vi "initindexstime.vi"(0 "object in":refnum<class "interface.lvclass">, 5 "error in (no error)":errorcluster) -> (14 "object out":refnum<class "interface.lvclass">, 19 "error out":errorcluster)   [LabVIEW 2016, in "interface.lvclass"]
uses:
  interface.lvclass
  <vilib>/Utility/config.llb/NI_LVConfig.lvlib
  <vilib>/Utility/config.llb/Read Key (String).vi
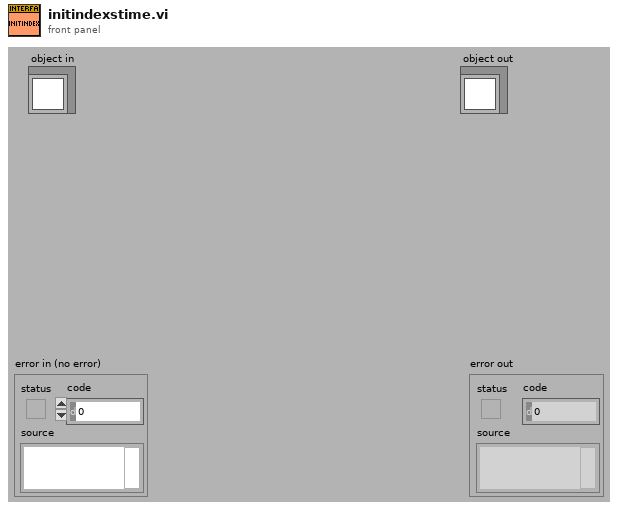
[diagram p1: front panel]
types:
  T1 = cluster{"CODMn":string, "CODCr":string, "DO":string, "铜":string, "PH":string, "氨氮":string, "比电导率":string, "水温":string, "COD":string, "浊度":string, "总氮":string, "总磷":string, "叶绿素a":string, "藻密度":string, "水位":string, "流速":string, "瞬时流量":string, "累积流量":string, "亚硝酸盐":string, "硫化物":string, "ORP":string, "铅":string, "镉":string, "锌":string, "镍":string, "锰":string, "汞":string, "气温":string, "气压":string, "风速":string, "风向":string, "盐度":string, "磷酸盐":string, "硝氮":string, "氟化物":string, "挥发酚":string, "氯化物":string}
  T2 = cluster{"氨氮仪器参数索引起始时间":string, "总磷仪器参数索引起始时间":string, "总氮仪器参数索引起始时间":string, "CODMn仪器参数索引起始时间":string, "CODCr仪器参数索引起始时间":string, "DO仪器参数索引起始时间":string, "PH仪器参数索引起始时间":string, "比电导率仪器参数索引起始时间":string, "水温仪器参数索引起始时间":string, "浊度仪器参数索引起始时间":string, "叶绿素a仪器参数索引起始时间":string, "藻密度仪器参数索引起始时间":string, "ORP仪器参数索引起始时间":string, "氟化物仪器参数索引起始时间":string, "挥发酚仪器参数索引起始时间":string}
  T3 = typedef "LVDateTimeRec.ctl" = cluster{"秒数的小数部分":dbl, "秒":i32, "分":i32, "时":i32, "日":i32, "月":i32, "年":i32, "天数（周）":i32, "天数（年）":i32, "DST":i32}
  T4 = cluster{"氨氮报警信息索引起始时间":string, "总磷报警信息索引起始时间":string, "总氮报警信息索引起始时间":string, "CODMn报警信息索引起始时间":string, "CODCr报警信息索引起始时间":string, "DO报警信息索引起始时间":string, "PH报警信息索引起始时间":string, "比电导率报警信息索引起始时间":string, "水温报警信息索引起始时间":string, "浊度报警信息索引起始时间":string, "叶绿素报警信息索引起始时间":string, "系统报警信息索引起始时间":string, "氟化物报警信息索引起始时间":string, "挥发酚报警信息索引起始时间":string}
  T5 = cluster{"氨氮零点核查索引起始时间":string, "总磷零点核查索引起始时间":string, "总氮零点核查索引起始时间":string, "CODMn零点核查索引起始时间":string, "CODCr零点核查索引起始时间":string, "亚硝酸盐零点核查索引起始时间":string, "硫化物零点核查索引起始时间":string, "ORP零点核查索引起始时间":string, "氟化物零点核查索引起始时间":string, "挥发酚零点核查索引起始时间":string}
  T6 = cluster{"氨氮加标回收索引起始时间":string, "总磷加标回收索引起始时间":string, "总氮加标回收索引起始时间":string, "CODMn加标回收索引起始时间":string, "CODCr加标回收索引起始时间":string, "氟化物加标回收索引起始时间":string, "挥发酚加标回收索引起始时间":string}
  T7 = cluster{"氨氮仪器日志索引起始时间":string, "总磷仪器日志索引起始时间":string, "总氮仪器日志索引起始时间":string, "CODMn仪器日志索引起始时间":string, "CODCr仪器日志索引起始时间":string, "系统仪器日志索引起始时间":string, "氟化物仪器日志索引起始时间":string, "挥发酚仪器日志索引起始时间":string}
  T8 = cluster{"氨氮跨度核查索引起始时间":string, "总磷跨度核查索引起始时间":string, "总氮跨度核查索引起始时间":string, "CODMn跨度核查索引起始时间":string, "CODCr跨度核查索引起始时间":string, "亚硝酸盐跨度核查索引起始时间":string, "硫化物跨度核查索引起始时间":string, "ORP跨度核查索引起始时间":string, "氟化物跨度核查索引起始时间":string, "挥发酚跨度核查索引起始时间":string}
  T9 = cluster{"氨氮集成干预索引起始时间":string, "总磷集成干预索引起始时间":string, "总氮集成干预索引起始时间":string, "CODMn集成干预索引起始时间":string, "CODCr集成干预索引起始时间":string, "DO集成干预索引起始时间":string, "PH集成干预索引起始时间":string, "比电导率集成干预索引起始时间":string, "水温集成干预索引起始时间":string, "浊度集成干预索引起始时间":string, "叶绿素a集成干预索引起始时间":string, "藻密度集成干预索引起始时间":string, "亚硝酸盐集成干预索引起始时间":string, "硫化物集成干预索引起始时间":string, "ORP集成干预索引起始时间":string, "氟化物集成干预索引起始时间":string, "挥发酚集成干预索引起始时间":string, "氯化物集成干预索引起始时间":string}
  T10 = cluster{"氨氮标样核查索引起始时间":string, "总磷标样核查索引起始时间":string, "总氮标样核查索引起始时间":string, "CODMn标样核查索引起始时间":string, "CODCr标样核查索引起始时间":string, "DO标样核查索引起始时间":string, "PH标样核查索引起始时间":string, "比电导率标样核查索引起始时间":string, "水温标样核查索引起始时间":string, "浊度标样核查索引起始时间":string, "叶绿素a标样核查索引起始时间":string, "藻密度标样核查索引起始时间":string, "亚硝酸盐标样核查索引起始时间":string, "硫化物标样核查索引起始时间":string, "ORP标样核查索引起始时间":string, "氟化物标样核查索引起始时间":string, "挥发酚标样核查索引起始时间":string, "氯化物标样核查索引起始时间":string}
  T11 = cluster{"氨氮平行样索引起始时间":string, "总磷平行样索引起始时间":string, "总氮平行样索引起始时间":string, "CODMn平行样索引起始时间":string, "CODCr平行样索引起始时间":string, "氟化物平行样索引起始时间":string, "挥发酚平行样索引起始时间":string}
  T12 = typedef "NI_LVConfig.lvlib/Config Data RefNum.ctl" = refnum<k1>
  T13 = cluster{"[0]":string, "[1]":string, "[2]":string, "[3]":string, "[4]":string, "[5]":string, "[6]":string, "[7]":string, "[8]":string, "[9]":string, "[10]":string, "[11]":string, "[12]":string, "[13]":string}
  T14 = cluster{"[0]":string, "[1]":string, "[2]":string, "[3]":string, "[4]":string, "[5]":string, "[6]":string, "[7]":string, "[8]":string, "[9]":string}
  T15 = cluster{"[0]":string, "[1]":string, "[2]":string, "[3]":string, "[4]":string, "[5]":string, "[6]":string, "[7]":string, "[8]":string, "[9]":string, "[10]":string, "[11]":string, "[12]":string, "[13]":string, "[14]":string}
  T16 = cluster{"[0]":string, "[1]":string, "[2]":string, "[3]":string, "[4]":string, "[5]":string, "[6]":string}
  T17 = cluster{"[0]":string, "[1]":string, "[2]":string, "[3]":string, "[4]":string, "[5]":string, "[6]":string, "[7]":string}
  T18 = cluster{"[0]":string, "[1]":string, "[2]":string, "[3]":string, "[4]":string, "[5]":string, "[6]":string, "[7]":string, "[8]":string, "[9]":string, "[10]":string, "[11]":string, "[12]":string, "[13]":string, "[14]":string, "[15]":string, "[16]":string, "[17]":string}
  T19 = cluster{"[0]":string, "[1]":string, "[2]":string, "[3]":string, "[4]":string, "[5]":string, "[6]":string, "[7]":string, "[8]":string, "[9]":string, "[10]":string, "[11]":string, "[12]":string, "[13]":string, "[14]":string, "[15]":string, "[16]":string, "[17]":string, "[18]":string, "[19]":string, "[20]":string, "[21]":string, "[22]":string, "[23]":string, "[24]":string, "[25]":string, "[26]":string, "[27]":string, "[28]":string, "[29]":string, "[30]":string, "[31]":string, "[32]":string, "[33]":string, "[34]":string, "[35]":string, "[36]":string}
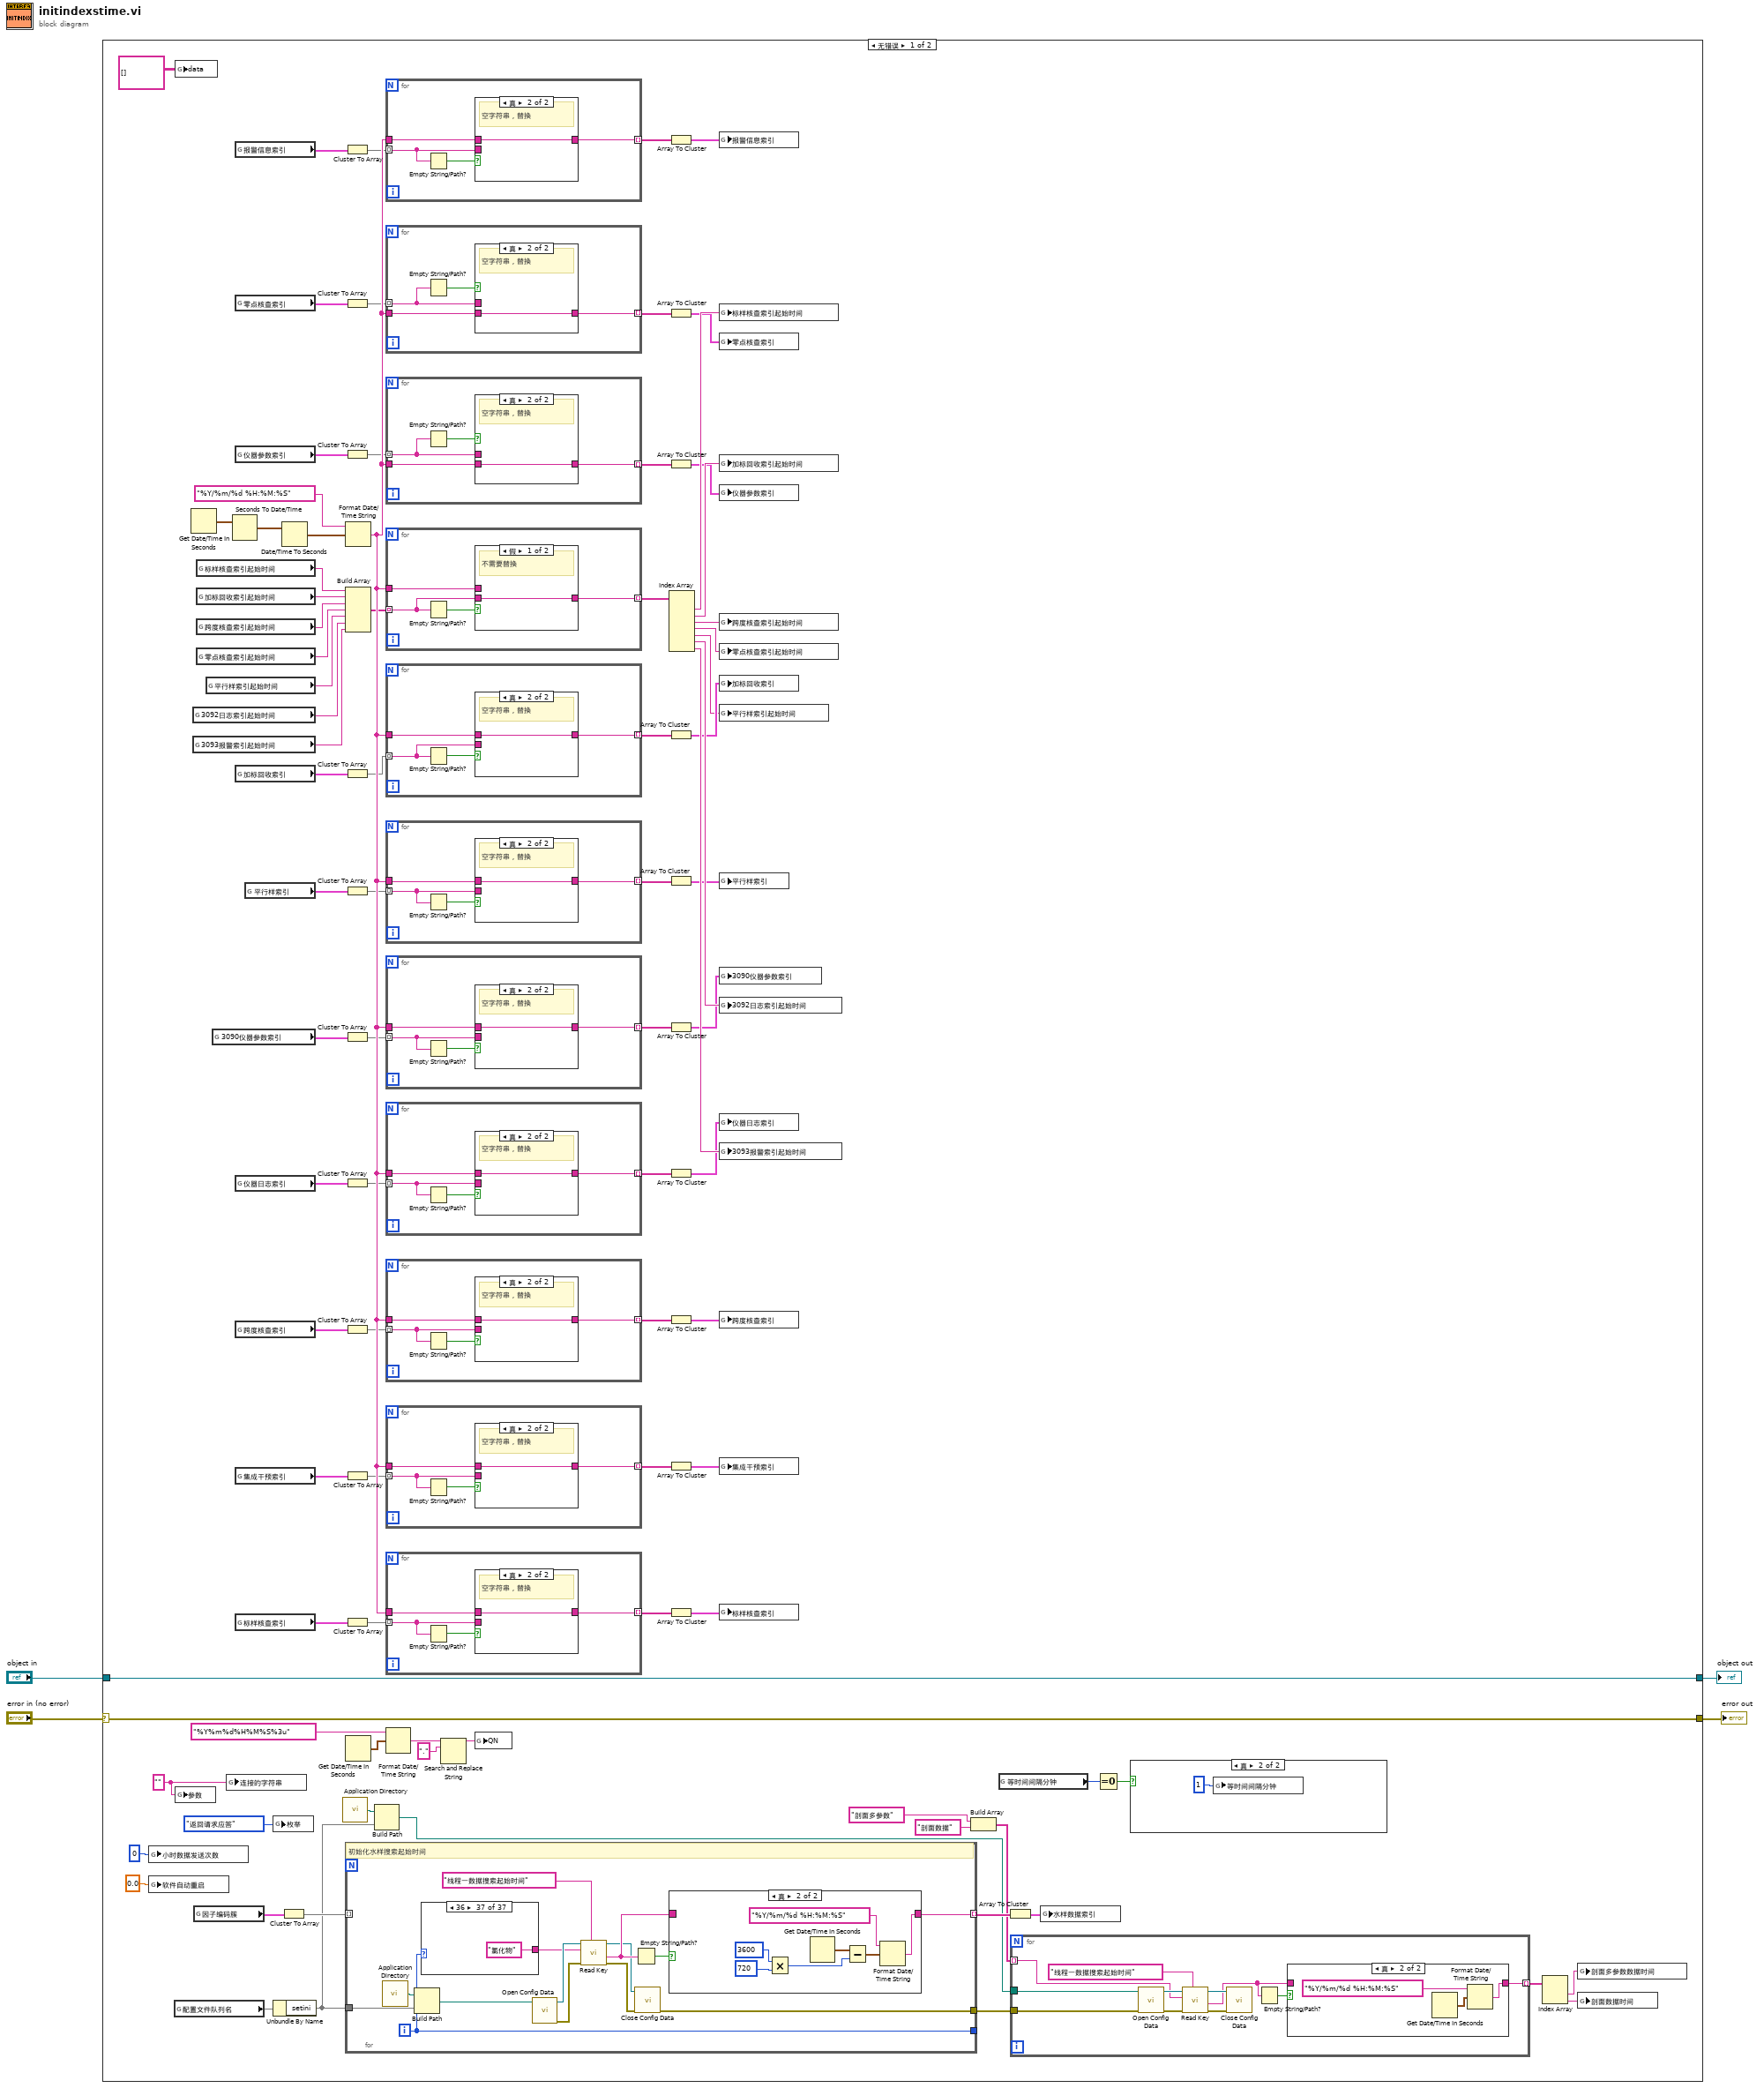
[diagram p0: block diagram]
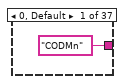
[diagram p5: hidden frame]
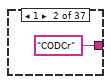
[diagram p6: hidden frame]
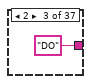
[diagram p7: hidden frame]
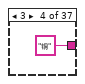
[diagram p8: hidden frame]
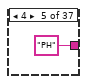
[diagram p9: hidden frame]
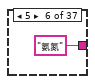
[diagram p10: hidden frame]
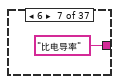
[diagram p11: hidden frame]
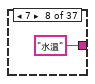
[diagram p12: hidden frame]
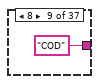
[diagram p13: hidden frame]
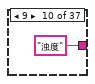
[diagram p14: hidden frame]
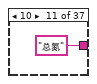
[diagram p15: hidden frame]
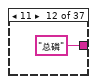
[diagram p16: hidden frame]
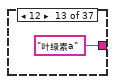
[diagram p17: hidden frame]
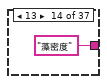
[diagram p18: hidden frame]
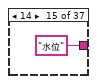
[diagram p19: hidden frame]
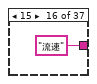
[diagram p20: hidden frame]
diagram:
  n1 = case shown="无错误" "error in (no error)" {
    selector: "error in (no error)" -> [w94 w237]
    tunnel: [w94 w237] -> w3
    tunnel: [w93 w236] -> w1
    tunnel: "object in" -> [w93 w236]
    frame No Error {
      w8 = "" ("参数")
      n2 = global write "全局 小时数据发送次数.vi" "小时数据发送次数"(0 ("数值")) -> ()
      n3 = global write "全局1.vi" "软件自动重启"(0.0 ("软件自动重启")) -> ()
      n4 = global read "断电保存全局.vi" "配置文件队列名"() -> (w24)
      n5 = global write "全局 实时数据参数.vi" "data"(string[][] [] ("data")) -> ()
      n6 = global write "全局 实时数据参数.vi" "参数"(w8) -> ()
      n7 = Get Date/Time In Seconds() -> (seconds since 1Jan1904=w32:timestamp)
      n8 = global read "全局 时间2.vi" "3092日志索引起始时间"() -> (w89:string)
      n9 = global read "全局 时间2.vi" "3093报警索引起始时间"() -> (w91:string)
      n10 = global read "断电保存全局.vi" "因子编码簇"() -> (w25:T1)
      n11 = global read "全局 时间2.vi" "标样核查索引起始时间"() -> (w68:string)
      n12 = global read "全局 时间2.vi" "加标回收索引起始时间"() -> (w69:string)
      n13 = global read "全局 时间2.vi" "跨度核查索引起始时间"() -> (w70:string)
      n14 = global read "全局 时间2.vi" "零点核查索引起始时间"() -> (w72:string)
      n15 = global read "全局 时间2.vi" "平行样索引起始时间"() -> (w71:string)
      n16 = global read "全局 时间2.vi" "3090仪器参数索引"() -> (w80:T2)
      n17 = global write "全局 实时数据参数.vi" "连接的字符串"(w8) -> ()
      n18 = Seconds To Date/Time(time stamp (now)=w32) -> (date time rec=w34:T3)  [unwired: 1 in]
      n19 = global read "全局 时间2.vi" "报警信息索引"() -> (w43:T4)
      n20 = global read "全局 时间2.vi" "零点核查索引"() -> (w36:T5)
      n21 = global read "全局 时间2.vi" "仪器参数索引"() -> (w63:T2)
      n22 = global read "全局 时间2.vi" "加标回收索引"() -> (w84:T6)
      n23 = global read "全局 时间2.vi" "仪器日志索引"() -> (w64:T7)
      n24 = global read "全局 时间2.vi" "跨度核查索引"() -> (w55:T8)
      n25 = global read "全局 时间2.vi" "集成干预索引"() -> (w51:T9)
      n26 = global read "全局 时间2.vi" "标样核查索引"() -> (w44:T10)
      n27 = global read "全局 时间2.vi" "平行样索引"() -> (w56:T11)
      n28 = global write "全局1.vi" "枚举"(enum16{"返回请求应答", "上传数据", "返回执行结果"}."返回请求应答" ("枚举")) -> ()
      n29 = Unbundle By Name(w24) -> ("setini"=w23)
      n30 = Cluster To Array(cluster=w25) -> (array=w31:string[])
      n31 = Date/Time To Seconds(2:w34) -> (0:w35:timestamp)  [unwired: 1 in]
      n32 = call <vilib>:"Application Directory.vi"() -> ("Application Directory"=w28:path)
      n33 = Cluster To Array(cluster=w43) -> (array=w42:string[])
      n34 = Cluster To Array(cluster=w36) -> (array=w37:string[])
      n35 = Cluster To Array(cluster=w63) -> (array=w62:string[])
      n36 = Cluster To Array(cluster=w84) -> (array=w85:string[])
      n37 = Cluster To Array(cluster=w56) -> (array=w57:string[])
      n38 = Cluster To Array(cluster=w80) -> (array=w81:string[])
      n39 = Cluster To Array(cluster=w64) -> (array=w65:string[])
      n40 = Cluster To Array(cluster=w55) -> (array=w54:string[])
      n41 = Cluster To Array(cluster=w51) -> (array=w50:string[])
      n42 = Cluster To Array(cluster=w44) -> (array=w45:string[])
      n43 = Format Date/Time String(time format string (%c)="%Y/%m/%d %H:%M:%S" ("时间格式字符串(%c)"), seconds (now)=w35) -> (date/time string=w88:string)  [unwired: 1 in]
      n44 = Build Array(w68, w69, w70, w72, w71, w89, w91) -> (w73:string[])
      n45 = Get Date/Time In Seconds() -> (seconds since 1Jan1904=w13:timestamp)
      n46 = for {
        tunnel: w31 -> [_] mode=indexing
        tunnel: [w116] -> _
        tunnel: [w113] -> w30 mode=indexing
        tunnel: [w112] -> w26
        tunnel: w23 -> [w111]
        i -> [w116]
        # "初始化水样搜索起始时间"
        n47 = call <vilib>:"Application Directory.vi"() -> ("Application Directory"=w124:path)
        n48 = Build Path(base path=w124, name or relative path=w111) -> (appended path=w123:path)
        n49 = case shown="36" w116 {
          tunnel: ["CODMn" "CODCr" "DO" "铜" "PH" "氨氮" "比电导率" "水温" "COD" "浊度" "总氮" "总磷" "叶绿素a" "藻密度" "水位" "流速" "瞬时流量" "累积流量" "亚硝氮" "硫化物" "ORP" "铅" "镉" "锌" "镍" "锰" "汞" "气温" "气压" "风速" "风向" "盐度" "磷酸盐" "硝氮" "氟化物" "挥发酚" "氯化物"] -> w119
          frame 0, Default {
          }
          frame 1 {
          }
          frame 2 {
          }
          frame 3 {
          }
          frame 4 {
          }
          frame 5 {
          }
          frame 6 {
          }
          frame 7 {
          }
          frame 8 {
          }
          frame 9 {
          }
          frame 10 {
          }
          frame 11 {
          }
          frame 12 {
          }
          frame 13 {
          }
          frame 14 {
          }
          frame 15 {
          }
          frame 16 {
          }
          frame 17 {
          }
          frame 18 {
          }
          frame 19 {
          }
          frame 20 {
          }
          frame 21 {
          }
          frame 22 {
          }
          frame 23 {
          }
          frame 24 {
          }
          frame 25 {
          }
          frame 26 {
          }
          frame 27 {
          }
          frame 28 {
          }
          frame 29 {
          }
          frame 30 {
          }
          frame 31 {
          }
          frame 32 {
          }
          frame 33 {
          }
          frame 34 {
          }
          frame 35 {
          }
          frame 36 {
          }
        }
        n50 = call <vilib>:"Open Config Data.vi"("configuration file path"=w123) -> ("error out"=w121:errorcluster, "refnum"=w122:T12)  [unwired: 8 in, 1 out]
        n51 = call-poly <vilib>:"Read Key.vi"("section"="线程一数据搜索起始时间", "error in (no error)"=w121, "key"=w119, "refnum"=w122) -> ("error out"=w114:errorcluster, "value"=w117:string, "refnum out"=w115:T12)  [unwired: 4 in, 1 out]
        n52 = Empty String/Path?(string/path=w117) -> (empty?=w118:bool)
        n53 = call <vilib>:"Close Config Data.vi"("error in (no error)"=w114, "refnum"=w115) -> ("error out"=w112:errorcluster)  [unwired: 8 in, 1 out]
        n54 = case shown="真" w118 {
          tunnel: [w125 w131] -> w113
          tunnel: w117 -> [w125 _]
          frame False {
          }
          frame True {
            n55 = Multiply(x=3600, y=720) -> (x*y=w127:i32)
            n56 = Get Date/Time In Seconds() -> (seconds since 1Jan1904=w130:timestamp)
            n57 = Subtract(x=w130, y=w127) -> (x-y=w126:timestamp)
            n58 = Format Date/Time String(time format string (%c)="%Y/%m/%d %H:%M:%S" ("时间格式字符串(%c)"), seconds (now)=w126) -> (date/time string=w131:string)  [unwired: 1 in]
          }
        }
      }
      n59 = Build Path(base path=w28, name or relative path=w23) -> (appended path=w27:path)
      n60 = for {
        tunnel: w42 -> [w224] mode=indexing
        tunnel: w88 -> [w226]
        tunnel: [w225] -> w41 mode=indexing
        n61 = Empty String/Path?(string/path=w224) -> (empty?=w227:bool)
        n62 = case shown="真" w227 {
          tunnel: w226 -> [_ w229]
          tunnel: [w228 w229] -> w225
          tunnel: w224 -> [w228 _]
          frame False {
            # "不需要替换"
          }
          frame True {
            # "空字符串，替换"
          }
        }
      }
      n63 = for {
        tunnel: w37 -> [w230] mode=indexing
        tunnel: w88 -> [w232]
        tunnel: [w231] -> w38 mode=indexing
        n64 = Empty String/Path?(string/path=w230) -> (empty?=w233:bool)
        n65 = case shown="真" w233 {
          tunnel: w232 -> [_ w235]
          tunnel: [w234 w235] -> w231
          tunnel: w230 -> [w234 _]
          frame False {
            # "不需要替换"
          }
          frame True {
            # "空字符串，替换"
          }
        }
      }
      n66 = for {
        tunnel: w62 -> [w194] mode=indexing
        tunnel: w88 -> [w196]
        tunnel: [w195] -> w61 mode=indexing
        n67 = Empty String/Path?(string/path=w194) -> (empty?=w197:bool)
        n68 = case shown="真" w197 {
          tunnel: w196 -> [_ w199]
          tunnel: [w198 w199] -> w195
          tunnel: w194 -> [w198 _]
          frame False {
            # "不需要替换"
          }
          frame True {
            # "空字符串，替换"
          }
        }
      }
      n69 = for {
        tunnel: w73 -> [w183] mode=indexing
        tunnel: w88 -> [w184]
        tunnel: [w182] -> w74 mode=indexing
        n70 = Empty String/Path?(string/path=w183) -> (empty?=w185:bool)
        n71 = case shown="假" w185 {
          tunnel: w184 -> [_ w187]
          tunnel: [w186 w187] -> w182
          tunnel: w183 -> [w186 _]
          frame False {
            # "不需要替换"
          }
          frame True {
            # "空字符串，替换"
          }
        }
      }
      n72 = for {
        tunnel: w85 -> [w170] mode=indexing
        tunnel: w88 -> [w172]
        tunnel: [w171] -> w86 mode=indexing
        n73 = Empty String/Path?(string/path=w170) -> (empty?=w173:bool)
        n74 = case shown="真" w173 {
          tunnel: w172 -> [_ w175]
          tunnel: [w174 w175] -> w171
          tunnel: w170 -> [w174 _]
          frame False {
            # "不需要替换"
          }
          frame True {
            # "空字符串，替换"
          }
        }
      }
      n75 = for {
        tunnel: w57 -> [w200] mode=indexing
        tunnel: w88 -> [w202]
        tunnel: [w201] -> w58 mode=indexing
        n76 = Empty String/Path?(string/path=w200) -> (empty?=w203:bool)
        n77 = case shown="真" w203 {
          tunnel: w202 -> [_ w205]
          tunnel: [w204 w205] -> w201
          tunnel: w200 -> [w204 _]
          frame False {
            # "不需要替换"
          }
          frame True {
            # "空字符串，替换"
          }
        }
      }
      n78 = for {
        tunnel: w81 -> [w176] mode=indexing
        tunnel: w88 -> [w178]
        tunnel: [w177] -> w82 mode=indexing
        n79 = Empty String/Path?(string/path=w176) -> (empty?=w179:bool)
        n80 = case shown="真" w179 {
          tunnel: w178 -> [_ w181]
          tunnel: [w180 w181] -> w177
          tunnel: w176 -> [w180 _]
          frame False {
            # "不需要替换"
          }
          frame True {
            # "空字符串，替换"
          }
        }
      }
      n81 = for {
        tunnel: w65 -> [w188] mode=indexing
        tunnel: w88 -> [w190]
        tunnel: [w189] -> w66 mode=indexing
        n82 = Empty String/Path?(string/path=w188) -> (empty?=w191:bool)
        n83 = case shown="真" w191 {
          tunnel: w190 -> [_ w193]
          tunnel: [w192 w193] -> w189
          tunnel: w188 -> [w192 _]
          frame False {
            # "不需要替换"
          }
          frame True {
            # "空字符串，替换"
          }
        }
      }
      n84 = for {
        tunnel: w54 -> [w206] mode=indexing
        tunnel: w88 -> [w208]
        tunnel: [w207] -> w53 mode=indexing
        n85 = Empty String/Path?(string/path=w206) -> (empty?=w209:bool)
        n86 = case shown="真" w209 {
          tunnel: w208 -> [_ w211]
          tunnel: [w210 w211] -> w207
          tunnel: w206 -> [w210 _]
          frame False {
            # "不需要替换"
          }
          frame True {
            # "空字符串，替换"
          }
        }
      }
      n87 = for {
        tunnel: w50 -> [w212] mode=indexing
        tunnel: w88 -> [w214]
        tunnel: [w213] -> w49 mode=indexing
        n88 = Empty String/Path?(string/path=w212) -> (empty?=w215:bool)
        n89 = case shown="真" w215 {
          tunnel: w214 -> [_ w217]
          tunnel: [w216 w217] -> w213
          tunnel: w212 -> [w216 _]
          frame False {
            # "不需要替换"
          }
          frame True {
            # "空字符串，替换"
          }
        }
      }
      n90 = for {
        tunnel: w45 -> [w218] mode=indexing
        tunnel: w88 -> [w220]
        tunnel: [w219] -> w46 mode=indexing
        n91 = Empty String/Path?(string/path=w218) -> (empty?=w221:bool)
        n92 = case shown="真" w221 {
          tunnel: w220 -> [_ w223]
          tunnel: [w222 w223] -> w219
          tunnel: w218 -> [w222 _]
          frame False {
            # "不需要替换"
          }
          frame True {
            # "空字符串，替换"
          }
        }
      }
      n93 = Format Date/Time String(time format string (%c)="%Y%m%d%H%M%S%3u" ("时间格式字符串(%c)"), seconds (now)=w13) -> (date/time string=w14:string)  [unwired: 1 in]
      n94 = Search and Replace String(input string=w14, search string="." ("搜索字符串")) -> (result string=w16:string)  [unwired: 6 in, 3 out]
      n95 = global write "全局1.vi" "QN"(w16) -> ()
      n96 = Array To Cluster(array=w41) -> (cluster=w40:T13)
      n97 = Array To Cluster(array=w38) -> (cluster=w39:T14)
      n98 = Array To Cluster(array=w61) -> (cluster=w60:T15)
      n99 = Array To Cluster(array=w86) -> (cluster=w87:T16)
      n100 = Array To Cluster(array=w58) -> (cluster=w59:T16)
      n101 = Array To Cluster(array=w82) -> (cluster=w83:T15)
      n102 = Array To Cluster(array=w66) -> (cluster=w67:T17)
      n103 = Array To Cluster(array=w53) -> (cluster=w52:T14)
      n104 = Array To Cluster(array=w49) -> (cluster=w48:T18)
      n105 = Array To Cluster(array=w46) -> (cluster=w47:T18)
      n106 = Index Array(array=w74) -> (element #1=w75:string, element #2=w76:string, element #3=w77:string, element #4=w79:string, element #5=w78:string, element #6=w90:string, element #7=w92:string)  [unwired: 7 in]
      n107 = global write "全局 时间2.vi" "报警信息索引"(w40) -> ()
      n108 = global write "全局 时间2.vi" "标样核查索引起始时间"(w75) -> ()
      n109 = global write "全局 时间2.vi" "零点核查索引"(w39) -> ()
      n110 = global write "全局 时间2.vi" "加标回收索引起始时间"(w76) -> ()
      n111 = global write "全局 时间2.vi" "仪器参数索引"(w60) -> ()
      n112 = global write "全局 时间2.vi" "跨度核查索引起始时间"(w77) -> ()
      n113 = global write "全局 时间2.vi" "零点核查索引起始时间"(w79) -> ()
      n114 = global write "全局 时间2.vi" "加标回收索引"(w87) -> ()
      n115 = global write "全局 时间2.vi" "平行样索引起始时间"(w78) -> ()
      n116 = global write "全局 时间2.vi" "平行样索引"(w59) -> ()
      n117 = global write "全局 时间2.vi" "3090仪器参数索引"(w83) -> ()
      n118 = global write "全局 时间2.vi" "3092日志索引起始时间"(w90) -> ()
      n119 = global write "全局 时间2.vi" "仪器日志索引"(w67) -> ()
      n120 = global write "全局 时间2.vi" "3093报警索引起始时间"(w92) -> ()
      n121 = global write "全局 时间2.vi" "跨度核查索引"(w52) -> ()
      n122 = global write "全局 时间2.vi" "集成干预索引"(w48) -> ()
      n123 = global write "全局 时间2.vi" "标样核查索引"(w47) -> ()
      n124 = Build Array("剖面多参数" ("key"), "剖面数据" ("key")) -> (w20:string[])
      n125 = global read "断电保存全局.vi" "等时间间隔分钟"() -> (w5:i32)
      n126 = Array To Cluster(array=w30) -> (cluster=w29:T19)
      n127 = for {
        tunnel: w27 -> [w106]
        tunnel: w26 -> [w105]
        tunnel: w20 -> [w97] mode=indexing
        tunnel: [w96] -> w19 mode=indexing
        n128 = call <vilib>:"Open Config Data.vi"("error in (no error)"=w105, "configuration file path"=w106) -> ("error out"=w102:errorcluster, "refnum"=w103:T12)  [unwired: 7 in, 1 out]
        n129 = call-poly <vilib>:"Read Key.vi"("section"="线程一数据搜索起始时间", "error in (no error)"=w102, "key"=w97, "refnum"=w103) -> ("error out"=w100:errorcluster, "value"=w99:string, "refnum out"=w101:T12)  [unwired: 4 in, 1 out]
        n130 = call <vilib>:"Close Config Data.vi"("error in (no error)"=w100, "refnum"=w101) -> ()  [unwired: 8 in, 2 out]
        n131 = Empty String/Path?(string/path=w99) -> (empty?=w98:bool)
        n132 = case shown="真" w98 {
          tunnel: [w107 w108] -> w96
          tunnel: w99 -> [w107 _]
          frame False {
          }
          frame True {
            n133 = Get Date/Time In Seconds() -> (seconds since 1Jan1904=w110:timestamp)
            n134 = Format Date/Time String(time format string (%c)="%Y/%m/%d %H:%M:%S" ("时间格式字符串(%c)"), seconds (now)=w110) -> (date/time string=w108:string)  [unwired: 1 in]
          }
        }
      }
      n135 = global write "全局 水样时间.vi" "水样数据索引"(w29) -> ()
      n136 = Equal To 0?(x=w5) -> (x = 0?=w6:bool)
      n137 = case shown="真" w6 {
        frame False {
        }
        frame True {
          n138 = global write "断电保存全局.vi" "等时间间隔分钟"(1 ("等时间间隔分钟")) -> ()
        }
      }
      n139 = Index Array(array=w19) -> (element #1=w18:string, element #2=w17:string)  [unwired: 2 in]
      n140 = global write "全局 水样时间.vi" "剖面多参数数据时间"(w18) -> ()
      n141 = global write "全局 水样时间.vi" "剖面数据时间"(w17) -> ()
    }
    frame Error {
    }
  }
  "error out" <- w3
  "object out" <- w1
